vi "Create Data Channel - Single Channel - Type Cast.vi"(8 "error in (no error)":errorcluster, 9 "settings":T1, 10 "channel name":string, 11 "response refnum in":T4 format="%.0x") -> (0 "error out":errorcluster, 2 "channel refnum":T4 format="%.0x", 3 "response refnum out":T4 format="%.0x")   [LabVIEW 2018, in "Instrument Addon Scripting API.lvlib"]
doc: "Creates a new Data Channel with the following configuration: \nData Type: Single Channel\nChannel Type: Type Cast\n\nInput: \nMessage Refnum In: reference to the \"Response\" message.\nName: represents the desired name of the channel.\nSettings: represents the settings applied on the new channel.\n\nOutput:\nMessage Refnum Out: reference to the \"Response\" message used as input.\nChannel Refnum: reference to the newly created channel."
uses:
  Instrument Addon Scripting API.lvlib
  <vilib>/NI Veristand/Custom Device API/Custom Device Item Ref.ctl
  TypeDefs/Single Channel Type Cast Settings.ctl
  Addon/Addon Shared/Types/Type Cast Type.ctl
  Addon/Addon Shared/Types/Endian.ctl
  Addon/Addon Shared/Types/Data Parameters.ctl
  Addon/Addon Shared/Types/Protocol Data Type.ctl
  Addon/Addon Shared/Types/Data Channel Type.ctl
  <vilib>/NI Veristand/Custom Device API/Custom Device Channel.ctl
  <vilib>/NI Veristand/Custom Device API/Custom Device Channel Type.ctl
  Addon/Addon Shared/Instrument Addon Shared.lvlib
  <vilib>/NI Veristand/Custom Device API/Custom Device API.lvlib
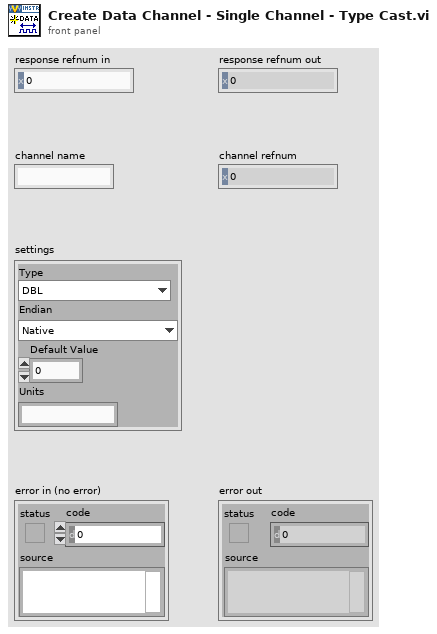
[diagram p1: front panel]
types:
  T1 = typedef "Instrument Addon Scripting API.lvlib/Single Channel Type Cast Settings.ctl" = cluster{"Type":T2, "Endian":T3, "Default Value":dbl, "Units":string}
  T2 = typedef "Instrument Addon Shared.lvlib/Type Cast Type.ctl" = enum16{"DBL", "SGL", "U64", "U32", "U16", "U8", "I64", "I32", "I16", "I8"}
  T3 = typedef "Instrument Addon Shared.lvlib/Endian.ctl" = enum16{"Native", "Little", "Big"}
  T4 = typedef "Custom Device API.lvlib/Custom Device Item Ref.ctl" = u64
  T5 = typedef "Instrument Addon Shared.lvlib/Data Channel Type.ctl" = enum16{"Format", "Comparison", "Type Cast", "Enumerated List"}
  T6 = typedef "Instrument Addon Shared.lvlib/Protocol Data Type.ctl" = enum16{"Single Channel", "Array"}
  T7 = typedef "Custom Device API.lvlib/Custom Device Channel.ctl" = cluster{"Type":T8, "Units":string, "Default Value":dbl, "Faultable":bool, "Scalable":bool}
  T8 = typedef "Custom Device API.lvlib/Custom Device Channel Type.ctl" = enum16{"Input", "Output"}
  T9 = typedef "Instrument Addon Shared.lvlib/Data Parameters.ctl" = cluster{"Data Type":T6, "Channel Type":T5, "Format String":string, "Expected String":string, "Type":T2, "List":string[], "Delimiter":string, "Endian":T3}
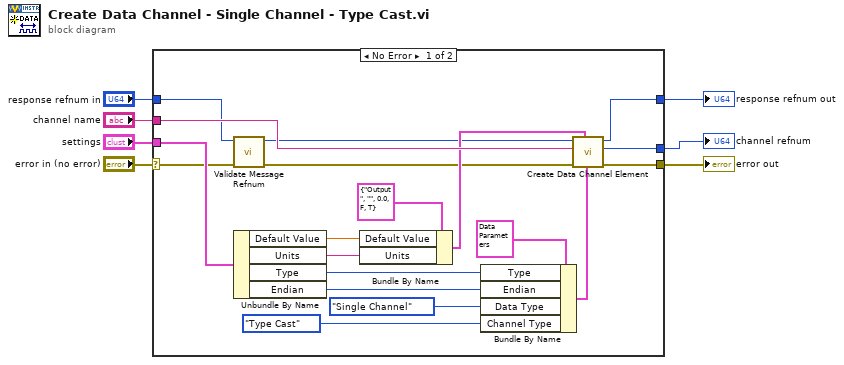
[diagram p0: block diagram]
diagram:
  n1 = case shown="No Error" "error in (no error)" {
    selector: "error in (no error)" -> [w11 w28]
    tunnel: [w16 w28] -> w7
    tunnel: [w13 w27] -> w6
    tunnel: "channel name" -> [w22 _]
    tunnel: "response refnum in" -> [w9 w27]
    tunnel: "settings" -> [w21 _]
    tunnel: [w12 _] -> w1
    frame No Error {
      n2 = call "Validate Message Refnum.vi"("error in (no error)"=w11, "Message in"=w9) -> ("error out"=w10:errorcluster, "Message out"=w8:T4)  [unwired: 8 in]
      n3 = Unbundle By Name(w21) -> ("Default Value"=w24:dbl, "Units"=w23:string, "Type"=w20:T2, "Endian"=w19:T3)
      n4 = Bundle By Name(cluster=T7 {"Type"=enum."Output", "Units"="", "Default Value"=0.0, "Faultable"=FALSE, "Scalable"=TRUE} ("Channel"), "Default Value"=w24, "Units"=w23) -> (w14:T7)
      n5 = Bundle By Name(cluster=T9 {"Data Type"=enum."Single Channel", "Channel Type"=enum."Format", "Format String"="%.3g", "Expected String"="", "Type"=enum."SGL", "List"=[], "Delimiter"=",", "Endian"=enum."Native"} ("Data Parameters"), "Type"=w20, "Endian"=w19, "Data Type"=Protocol_Data_Type."Single Channel", "Channel Type"=Data_Channel_Type."Type Cast") -> (w15:T9)
      n6 = call "Create Data Channel Element.vi"("Data Channel Parameters"=w15, "Settings"=w14, "Error In"=w10, "Name"=w22, "Refnum In"=w8) -> ("Error Out"=w16:errorcluster, "Channel Refnum"=w12:T4, "Refnum Out"=w13:T4)  [unwired: 4 in]
    }
    frame Error {
    }
  }
  "error out" <- w7
  "response refnum out" <- w6
  "channel refnum" <- w1
